vi "ICM Interpolate Arrays.vi"(8 "Mode (Advanced)":bool=TRUE, 9 "Scaled Array":dbl[](array[numeric]), 10 "Raw Array":dbl[](array[numeric]), 11 "Data In":dbl) -> (3 "Data Out":dbl)   [LabVIEW 2024]
doc: "ICM Interpolate Arrays.vi\n\nThis VI is used to scale a raw data value according to a lookup table. The \"Basic\" mode uses straight linear interpolation using built-in LabVIEW functions. Note that input values above or below the Raw Value array range will peg at the maximum or minimum Scaled values. The \"Advanced\" mode (which is default) finds the nearest 5 points and fits them to a second order polynomial, which is then extrapolated to the desired value. This allows for decent interpolation above and below the range of the arrays as well as improved accuracy within the ranges of the arrays.\n\nOriginal Code by David Thomson www.originalcode.com October, 2012\n\ncopyright 2012, Original Code Consulting"
uses:
  <vilib>/Analysis/NI_AALPro.lvlib
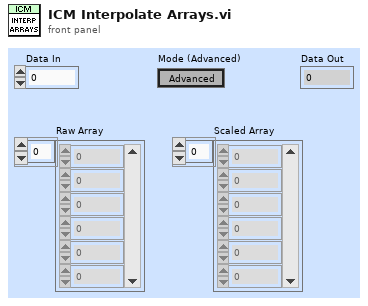
[diagram p1: front panel]
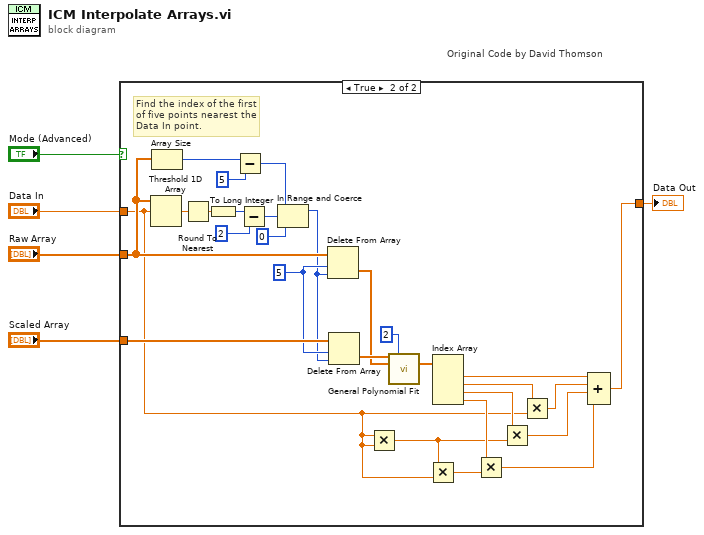
[diagram p0: block diagram]
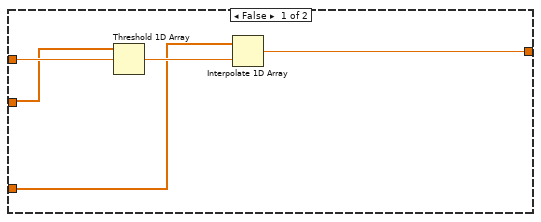
[diagram p2: hidden frame]
diagram:
  n1 = case "Original Code by David Thomson" shown="True" "Mode (Advanced)" {
    tunnel: "Data In" -> [w9 w11]
    tunnel: "Raw Array" -> [w8 w29]
    tunnel: "Scaled Array" -> [w7 w28]
    tunnel: [w6 w20] -> w1
    frame False {
      n2 = Threshold 1D Array(2:w9, 3:w8) -> (0:w10:dbl)  [unwired: 1 out]
      n3 = Interpolate 1D Array(1:w10, 2:w7) -> (0:w6:dbl)
    }
    frame True {
      w27 = 5 ("y")
      # "Find the index of the first\nof five points nearest the\nData In point."
      n4 = Threshold 1D Array(2:w11, 3:w29) -> (0:w38:dbl)  [unwired: 1 out]
      n5 = Array Size(array=w29) -> (size(s)=w32:i32)
      n6 = Round To Nearest(number=w38) -> (nearest integer value=w37:dbl)
      n7 = To Long Integer(number=w37) -> (32bit integer=w35:i32)
      n8 = Subtract(x=w32, y=5) -> (x-y=w30:i32)
      n9 = Subtract(x=w35, y=2) -> (x-y=w34:i32)
      n10 = In Range and Coerce(upper limit=w30, x=w34, lower limit=0 ("y")) -> (coerced(x)=w26:i32)  [unwired: 1 out]
      n11 = Delete From Array(array=w29, length=w27, index=w26) -> (deleted portion=w23:dbl[])  [unwired: 1 out]
      n12 = Delete From Array(array=w28, length=w27, index=w26) -> (deleted portion=w24:dbl[])  [unwired: 1 out]
      n13 = Multiply(x=w11, y=w11) -> (x*y=w12:dbl)
      n14 = call <vilib>:"General Polynomial Fit.vi"("Y"=w24, "polynomial order"=2, "X"=w23) -> ("Polynomial Coefficients"=w22:dbl[])  [unwired: 9 in, 3 out]
      n15 = Multiply(x=w12, y=w11) -> (x*y=w13:dbl)
      n16 = Index Array(array=w22) -> (element #1=w21:dbl, element #2=w19:dbl, element #3=w17:dbl, element #4=w15:dbl)  [unwired: 4 in]
      n17 = Multiply(x=w15, y=w13) -> (x*y=w14:dbl)
      n18 = Multiply(x=w17, y=w12) -> (x*y=w16:dbl)
      n19 = Multiply(x=w19, y=w11) -> (x*y=w18:dbl)
      n20 = Compound Arithmetic op=ADD(w21, w18, w16, w14) -> (w20:dbl)
    }
  }
  "Data Out" <- w1
